vi "Angle Mag To RGB.vi"(8 "Magnitude (0-1)":dbl, 11 "Angle (Degrees)":dbl) -> (0 "RGB Color":u32(colorbox), 1 "Blue":u8, 2 "Green":u8, 3 "Red":u8)   [LabVIEW 2011, in "LabVIEW Interface for Arduino.lvlib"]
doc: "Converts an angle in degrees and a magnitude (0 to 1) to an RGB color."
uses:
  LabVIEW Interface for Arduino.lvlib
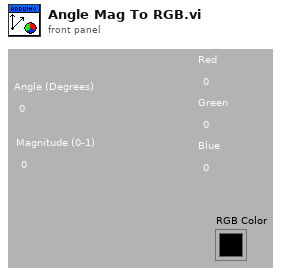
[diagram p1: front panel]
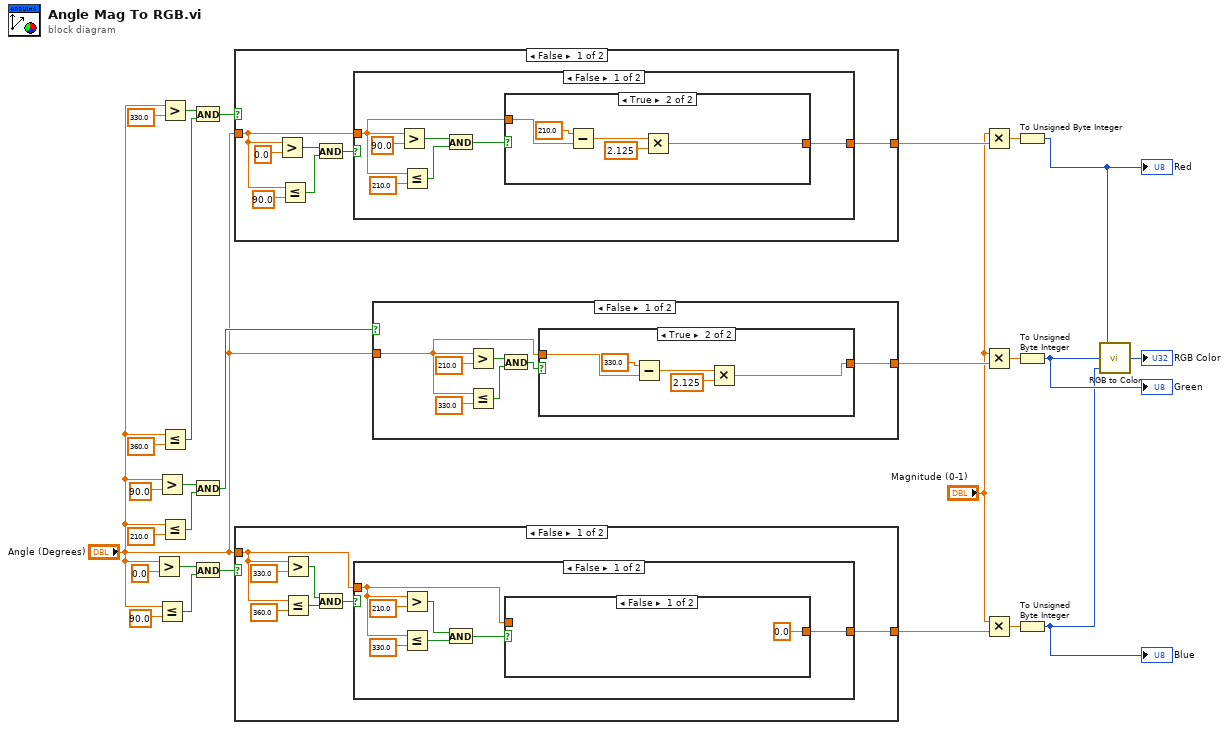
[diagram p0: block diagram]
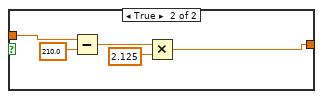
[diagram p2: hidden frame]
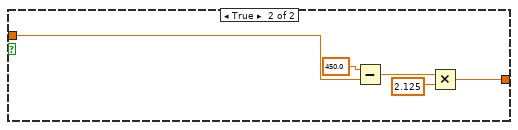
[diagram p3: hidden frame]
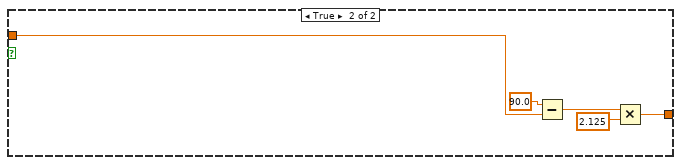
[diagram p4: hidden frame]
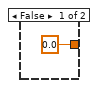
[diagram p5: hidden frame]
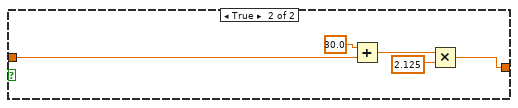
[diagram p6: hidden frame]
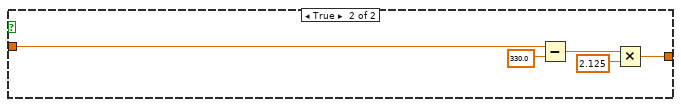
[diagram p7: hidden frame]
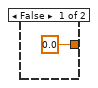
[diagram p8: hidden frame]
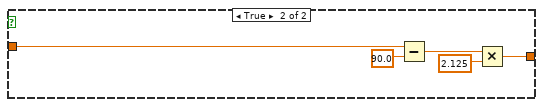
[diagram p9: hidden frame]
diagram:
  n1 = Greater?(x="Angle (Degrees)", y=0.0) -> (0:w17:bool)
  n2 = Greater?(x="Angle (Degrees)", y=90.0) -> (0:w27:bool)
  n3 = Less Or Equal?(x="Angle (Degrees)", y=90.0) -> (x <= y?=w16:bool)
  n4 = Greater?(x="Angle (Degrees)", y=330.0) -> (0:w18:bool)
  n5 = Less Or Equal?(x="Angle (Degrees)", y=360.0) -> (x <= y?=w22:bool)
  n6 = Less Or Equal?(x="Angle (Degrees)", y=210.0) -> (x <= y?=w26:bool)
  n7 = And(x=w18, y=w22) -> (x .and. y?=w19:bool)
  n8 = And(x=w27, y=w26) -> (x .and. y?=w23:bool)
  n9 = And(x=w17, y=w16) -> (x .and. y?=w15:bool)
  n10 = case shown="False" w19 {
    tunnel: "Angle (Degrees)" -> [w29 w55]
    tunnel: [w28 w53] -> w10
    frame False {
      n11 = Greater?(x=w29, y=0.0) -> (0:w31:bool)
      n12 = Less Or Equal?(x=w29, y=90.0) -> (x <= y?=w34:bool)
      n13 = And(x=w31, y=w34) -> (x .and. y?=w30:bool)
      n14 = case shown="False" w30 {
        tunnel: w29 -> [w36 w49]
        tunnel: [w35 w48] -> w28
        frame False {
          n15 = Greater?(x=w36, y=90.0) -> (0:w41:bool)
          n16 = Less Or Equal?(x=w36, y=210.0) -> (x <= y?=w40:bool)
          n17 = And(x=w41, y=w40) -> (x .and. y?=w37:bool)
          n18 = case shown="True" w37 {
            tunnel: w36 -> [_ w44]
            tunnel: [0.0 w43] -> w35
            frame False {
            }
            frame True {
              n19 = Subtract(x=210.0 ("y"), y=w44) -> (x-y=w45:dbl)
              n20 = Multiply(x=w45, y=2.125) -> (x*y=w43:dbl)
            }
          }
        }
        frame True {
          n21 = Add(x=30.0 ("y"), y=w49) -> (x+y=w50:dbl)
          n22 = Multiply(x=w50, y=2.125) -> (x*y=w48:dbl)
        }
      }
    }
    frame True {
      n23 = Subtract(x=w55, y=330.0) -> (x-y=w56:dbl)
      n24 = Multiply(x=w56, y=2.125) -> (x*y=w53:dbl)
    }
  }
  n25 = case shown="False" w15 {
    tunnel: "Angle (Degrees)" -> [w59 w84]
    tunnel: [w58 w83] -> w12
    frame False {
      n26 = Greater?(x=w59, y=330.0) -> (0:w63:bool)
      n27 = Less Or Equal?(x=w59, y=360.0) -> (x <= y?=w64:bool)
      n28 = And(x=w63, y=w64) -> (x .and. y?=w60:bool)
      n29 = case shown="False" w60 {
        tunnel: w59 -> [w66 w79]
        tunnel: [w65 w78] -> w58
        frame False {
          n30 = Greater?(x=w66, y=210.0) -> (0:w71:bool)
          n31 = Less Or Equal?(x=w66, y=330.0) -> (x <= y?=w70:bool)
          n32 = And(x=w71, y=w70) -> (x .and. y?=w67:bool)
          n33 = case shown="False" w67 {
            tunnel: w66 -> [_ w75]
            tunnel: [0.0 w73] -> w65
            frame False {
            }
            frame True {
              n34 = Subtract(x=w75, y=210.0) -> (x-y=w77:dbl)
              n35 = Multiply(x=w77, y=2.125) -> (x*y=w73:dbl)
            }
          }
        }
        frame True {
          n36 = Subtract(x=450.0 ("y"), y=w79) -> (x-y=w82:dbl)
          n37 = Multiply(x=w82, y=2.125) -> (x*y=w78:dbl)
        }
      }
    }
    frame True {
      n38 = Subtract(x=90.0 ("y"), y=w84) -> (x-y=w87:dbl)
      n39 = Multiply(x=w87, y=2.125) -> (x*y=w83:dbl)
    }
  }
  n40 = case shown="False" w23 {
    tunnel: "Angle (Degrees)" -> [w88 w105]
    tunnel: [w89 w101] -> w9
    frame False {
      n41 = Greater?(x=w88, y=210.0) -> (0:w93:bool)
      n42 = Less Or Equal?(x=w88, y=330.0) -> (x <= y?=w94:bool)
      n43 = And(x=w93, y=w94) -> (x .and. y?=w90:bool)
      n44 = case shown="True" w90 {
        tunnel: [0.0 w98] -> w89
        tunnel: w88 -> [_ w97]
        frame False {
        }
        frame True {
          n45 = Subtract(x=330.0 ("y"), y=w97) -> (x-y=w100:dbl)
          n46 = Multiply(x=w100, y=2.125) -> (x*y=w98:dbl)
        }
      }
    }
    frame True {
      n47 = Subtract(x=w105, y=90.0) -> (x-y=w103:dbl)
      n48 = Multiply(x=w103, y=2.125) -> (x*y=w101:dbl)
    }
  }
  n49 = Multiply(x="Magnitude (0-1)", y=w10) -> (x*y=w7:dbl)
  n50 = Multiply(x="Magnitude (0-1)", y=w9) -> (x*y=w8:dbl)
  n51 = Multiply(x="Magnitude (0-1)", y=w12) -> (x*y=w11:dbl)
  n52 = To Unsigned Byte Integer(number=w7) -> (unsigned 8bit integer=w3:u8)
  "Red" <- w3
  n53 = To Unsigned Byte Integer(number=w8) -> (unsigned 8bit integer=w2:u8)
  "Green" <- w2
  n54 = To Unsigned Byte Integer(number=w11) -> (unsigned 8bit integer=w1:u8)
  "Blue" <- w1
  n55 = call <vilib>:"RGB to Color.vi"("B"=w1, "G"=w2, "R"=w3) -> ("Color"=→"RGB Color":u32)
